vi "PLC_Selector_ReadBool.vi"() -> ()   [LabVIEW 2017]
panel:
  out "Boolean":bool
  in  "PLC Type":i32
  in  "MemoryNumber":string
  in  "PLC Address":string
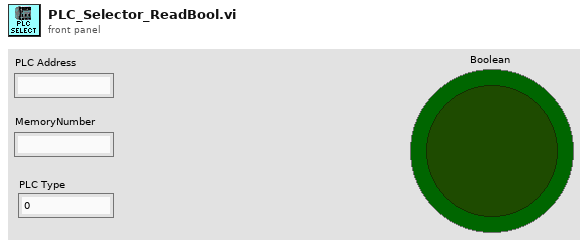
[diagram p1: front panel]
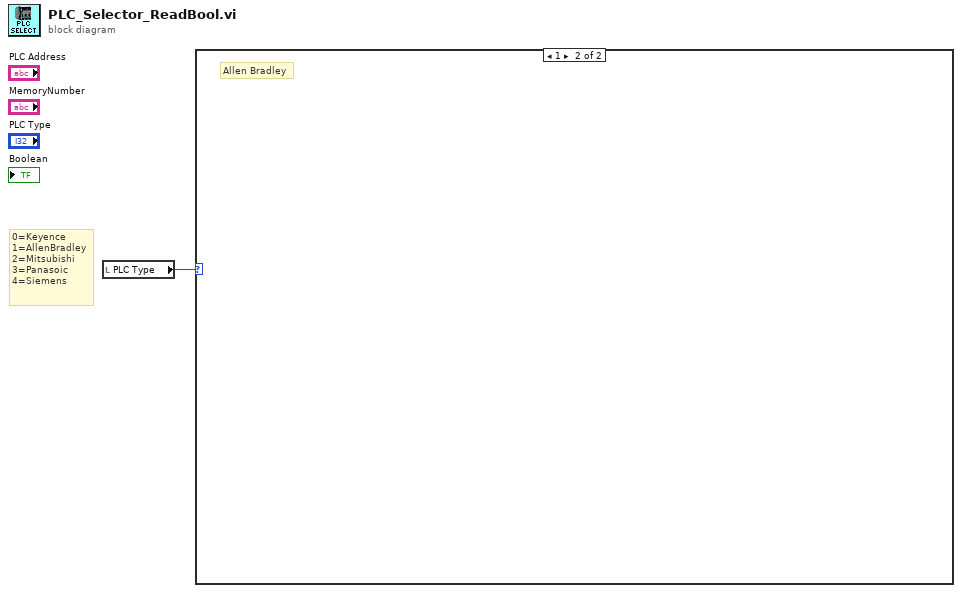
[diagram p0: block diagram]
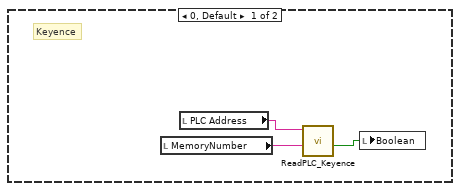
[diagram p2: hidden frame]
diagram:
  # "0=Keyence\n1=AllenBradley\n2=Mitsubishi\n3=Panasoic\n4=Siemens"
  n1 = local read "PLC Type"() -> (w1:i32)
  n2 = case shown="1" w1 {
    frame 0, Default {
      # "Keyence"
      n3 = local read "MemoryNumber"() -> (w3:string)
      n4 = local read "PLC Address"() -> (w4:string)
      n5 = call "ReadPLC_Keyence.vi"("MemoryNumber"=w3, "IP Address"=w4) -> ("BoolRead"=w2:bool)  [unwired: 9 in]
      n6 = local write "Boolean"(w2) -> ()
    }
    frame 1 {
      # "Allen Bradley"
    }
  }
